vi "Configure Standard Waveform.vi"(6 "DC Offset (0.00 V)":dbl, 7 "Frequency (1000 Hz)":dbl=1000.0, 8 "error in (no error)":errorcluster, 9 "Amplitude (1.0 Vpp)":dbl=1.0, 10 "Waveform Function (0: Sine)":u16(ring) items=["Sine", "Square", "Triangle"], 11 "VISA resource name":refnum<visa-resource-name>) -> (0 "error out":errorcluster, 3 "VISA resource name out":refnum<visa-resource-name>)   [LabVIEW 2013, in "Template - Function Generator.lvlib"]
doc: "Selects the waveform shape, frequency, amplitude, offset, and phase for a standard waveform."
uses:
  <instrlib>/_Template - Function Generator/Template - Function Generator.lvlib
panel:
  # "EDIT: If you have a  multi-channel function generators, add a channel control to this and all other channel-based VIs in the driver."
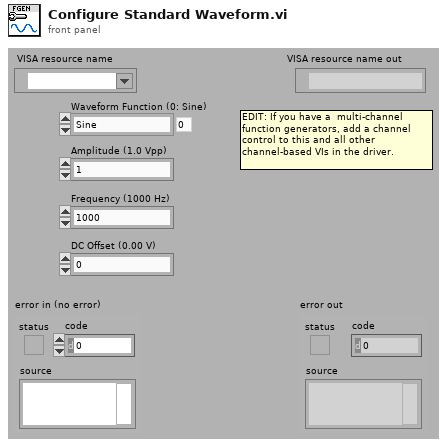
[diagram p1: front panel]
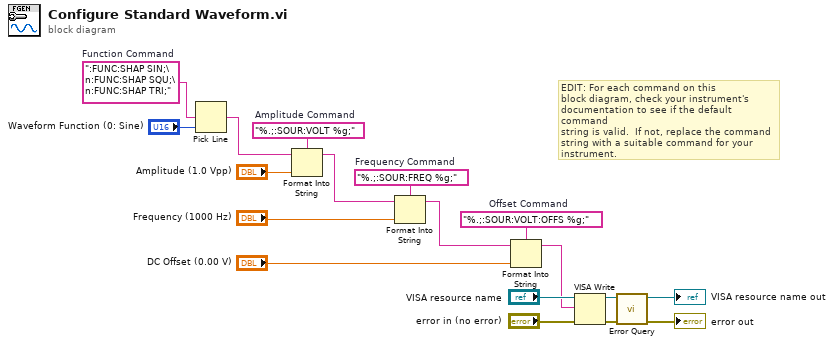
[diagram p0: block diagram]
diagram:
  w9 = "%.;:SOUR:VOLT:OFFS %g;"  # Offset Command
  w3 = "%.;:SOUR:VOLT %g;"  # Amplitude Command
  w4 = "%.;:SOUR:FREQ %g;"  # Frequency Command
  w11 = ":FUNC:SHAP SIN;\n:FUNC:SHAP SQU;\n:FUNC:SHAP TRI;"  # Function Command
  # "EDIT: For each command on this\nblock diagram, check your instrument's\ndocumentation to see if the default command\nstring is valid.  If not, replace the command\nstring with a suitable command for your\ninstrument."
  n1 = Pick Line(multi-line string=w11, line index="Waveform Function (0: Sine)") -> (output string=w10:string)  [unwired: 1 in]
  n2 = Format Into String(format string=w3, initial string=w10, "Amplitude (1.0 Vpp)") -> (resulting string=w6:string)  [unwired: 1 in, 1 out]
  n3 = Format Into String(format string=w4, initial string=w6, "Frequency (1000 Hz)") -> (resulting string=w7:string)  [unwired: 1 in, 1 out]
  n4 = Format Into String(format string=w9, initial string=w7, "DC Offset (0.00 V)") -> (resulting string=w5:string)  [unwired: 1 in, 1 out]
  n5 = VISA Write(VISA resource name="VISA resource name", write buffer=w5, error in (no error)="error in (no error)") -> (VISA resource name out=w14:refnum<visa-resource-name>, error out=w13:errorcluster)  [unwired: 1 out]
  n6 = call <instrlib>:"Error Query.vi"("error in (no error)"=w13, "VISA resource name"=w14) -> ("error out"=→"error out":errorcluster, "VISA resource name out"=→"VISA resource name out":refnum<visa-resource-name>)  [unwired: 6 in, 2 out]
